vi "Setup.vi"(8 "error in (no error)":errorcluster, 11 "XML Report Test In":refnum<class "Report Generator Test.lvclass">) -> (0 "error out":errorcluster, 3 "XML Report Test Out":refnum<class "Report Generator Test.lvclass">)   [LabVIEW 2020, in "Report Generator Test.lvclass"]
doc: "Setup method called by the testing framework before each test method is called."
uses:
  Report Generator Test.lvclass
  Report Generator Test.lvclass/Report Generator Test.ctl
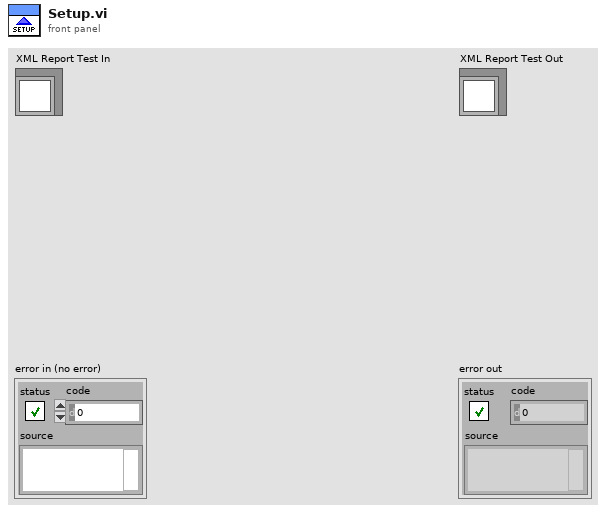
[diagram p1: front panel]
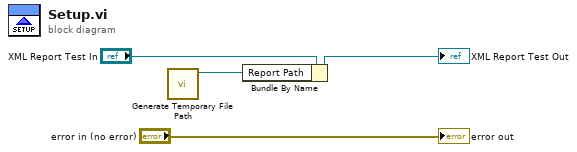
[diagram p0: block diagram]
diagram:
  n1 = call <vilib>:"Generate Temporary File Path.vi"() -> ("Unique Temporary File Path"=w1:path)  [unwired: 10 in, 1 out]
  n2 = Bundle By Name(cluster="XML Report Test In", "Report Path"=w1) -> (→"XML Report Test Out":refnum<class "Report Generator Test.lvclass">)
  "error out" <- "error in (no error)"
